vi "CSC_GetJointCoordInGCS.vi"(8 "error in (no error)":errorcluster, 11 "C-Alex in":refnum<class "CableSerialChain.lvclass">) -> (0 "error out":errorcluster, 1 "Jcoord & End Eff in GCS":dbl[][](array[numeric]), 2 "Joint Coord in GCS":dbl[][](array[numeric]), 3 "C-Alex out":refnum<class "CableSerialChain.lvclass">)   [LabVIEW 2015, in "CableSerialChain.lvclass"]
uses:
  CableSerialChain.lvclass
  Body/xyzO.ctl
  Body/Bodies.lvclass/Bodies.ctl
  CableSerialChain.lvclass/CableSerialChain.ctl
  <vilib>/Analysis/BLAS.llb/gemv - General Matrix-Vector Product.vi
  <vilib>/Analysis/BLAS.llb/dgemv - General Matrix-Vector Product (DBL).vi
  <vilib>/Utility/error.llb/Error Cluster From Error Code.vi
  Body/Bodies.lvclass
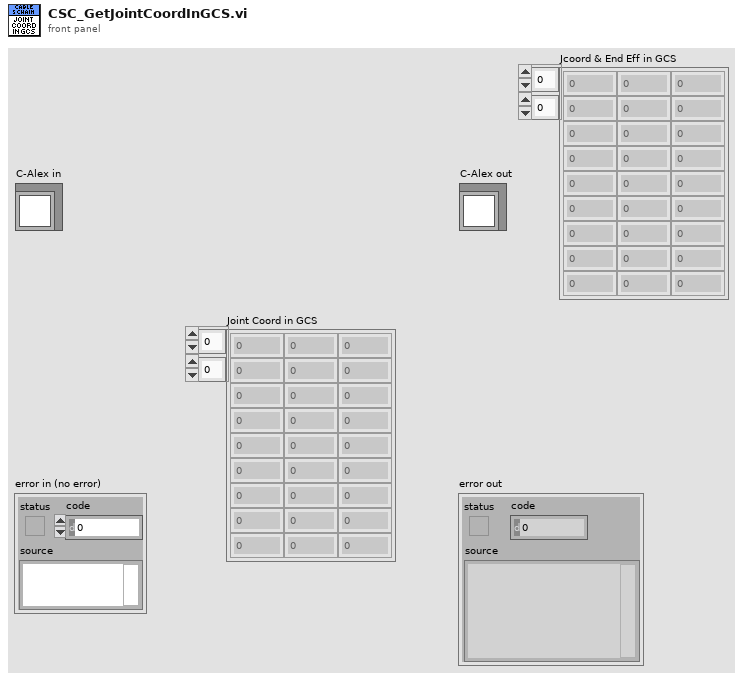
[diagram p1: front panel]
types:
  T1 = typedef "Bodies.lvclass/xyzO.ctl" = enum16{"X", "Y", "Z", "O"}
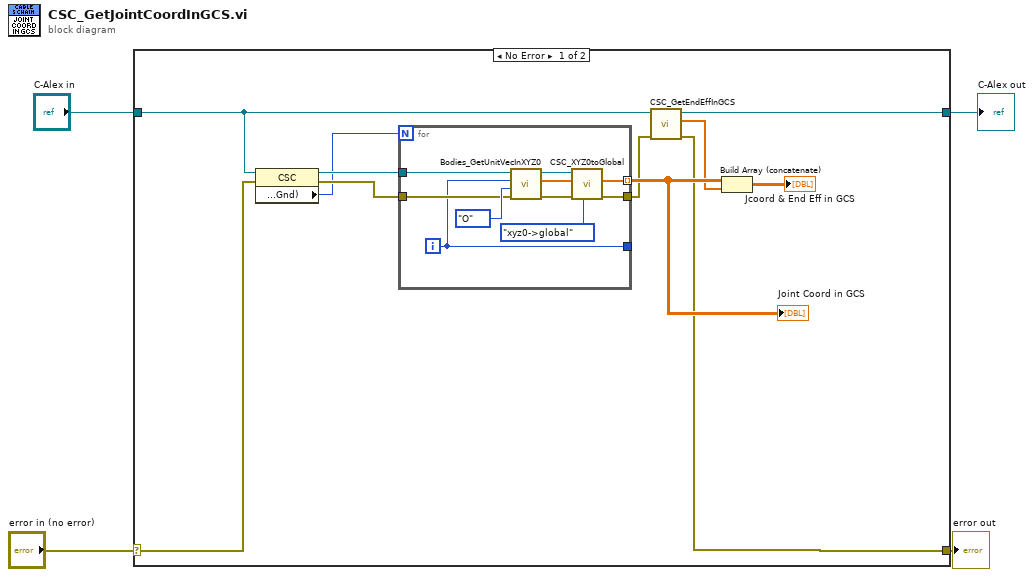
[diagram p0: block diagram]
diagram:
  n1 = case shown="No Error" "error in (no error)" {
    selector: "error in (no error)" -> [w15 w26]
    tunnel: [w8 w26] -> w3
    tunnel: [w12 w27] -> w1
    tunnel: "C-Alex in" -> [w5 w27]
    frame No Error {
      n2 = property class="CSC"(reference=w5, error in=w15) -> (reference out=w14:refnum<class "CableSerialChain.lvclass">, error out=w13:errorcluster, "#ofBodies(Inc.Gnd)"=w6:i32)
      n3 = for {
        N: w6 -> [_]
        tunnel: [w18] -> w11 mode=indexing
        tunnel: w14 -> [w25]
        tunnel: [w22] -> _
        tunnel: w13 -> [w23]
        tunnel: [w19] -> w9
        i -> [w22]
        n4 = call "Bodies_GetUnitVecInXYZ0.vi"("error in (no error)"=w23, "Dir of Vector"=xyzO."O" ("Dir"), "Body ID"=w22, "Bodies.lvclass"=w25) -> ("error out"=w20:errorcluster, "UnitVec in GCS"=w21:dbl[], "Bodies.lvclass 2"=w16:refnum<class "CableSerialChain.lvclass">)  [unwired: 5 in]
        n5 = call "CSC_XYZ0toGlobal.vi"("Dir(xyz0->global)"=enum16{"global->xyz0", "xyz0->global"}."xyz0->global" ("Dir"), "error in (no error)"=w20, "Pin"=w21, "CSC In"=w16) -> ("error out"=w19:errorcluster, "Pout"=w18:dbl[])  [unwired: 4 in, 2 out]
      }
      "Joint Coord in GCS" <- w11
      n6 = call "CSC_GetEndEffInGCS.vi"("error in (no error)"=w9, "CSC in"=w5) -> ("error out"=w8:errorcluster, "EndEffInGCS"=w7:dbl[], "CSC out"=w12:refnum<class "CableSerialChain.lvclass">)  [unwired: 5 in, 2 out]
      n7 = Build Array (concatenate)(w11, w7) -> (→"Jcoord & End Eff in GCS":dbl[][])
    }
    frame Error {
    }
  }
  "error out" <- w3
  "C-Alex out" <- w1
